vi "ImportedVideoConversion-CSV.vi"() -> ()   [LabVIEW 2019]
uses:
  RGB_To_Gray DLL Project/Project RGBToGray VI/RGBToGray.dll
  Gray_To_RGB DLL Project/Project Library For VI/Gray_to_RGB.dll
panel:
  out "Numeric":i32
  out "Frame Data":T1
  out "Elapsed time for Gray in sec":dbl
  out "RGB Frame":T2(plugin-control)
  out "Gray Frame":T2(plugin-control)
  in  "CSV File Path 2":path
  out "Elapsed time for RGB in sec":dbl
  out "Original Frame":T2(plugin-control)
  in  "Available Colormaps":T3
  in  "Stop":bool
  out "Progress Bar":i32(slide) max=677 scale=-1.0..677.0
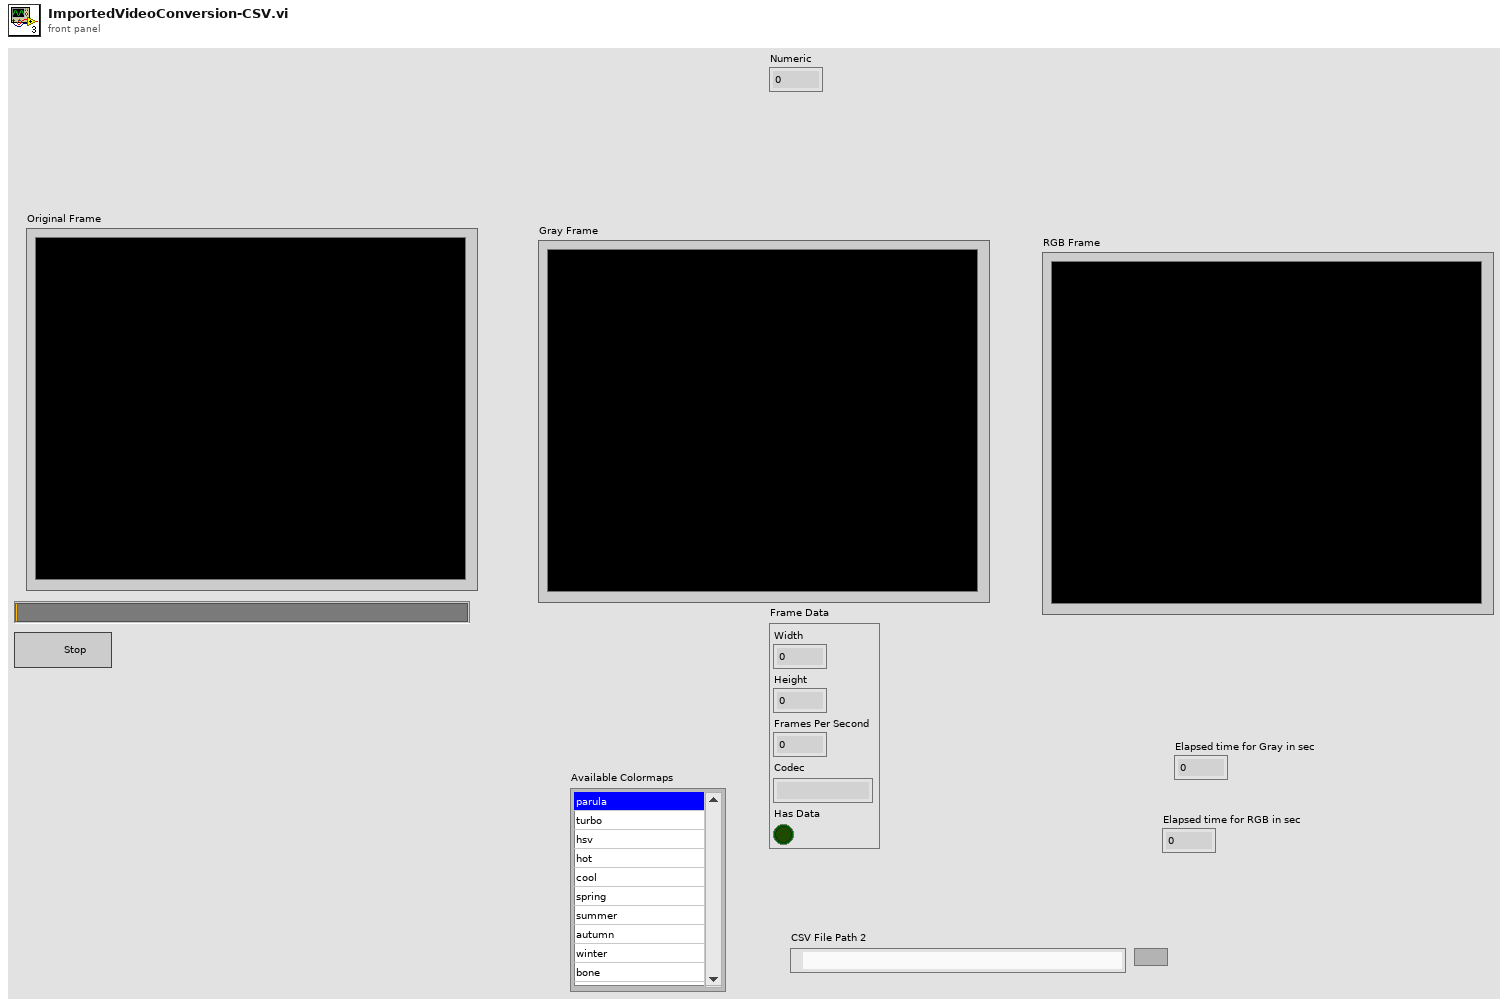
[diagram p1: front panel]
types:
  T1 = cluster{"Width":u32, "Height":u32, "Frames Per Second":u32, "Codec":string, "Has Data":bool}
  T2 = typedef "IMAQ Image.ctl" = refnum<image>
  T3 = typedef "Control 1.ctl" = i32
  T4 = typedef "Image Type" = u32
  T5 = typedef "IMAQ AVI2 Refnum.ctl" = refnum<k20>
  T6 = enum32{"Map Pixel Pointer", "Unmap Pixel Pointer", "Get Pixels Infos"}
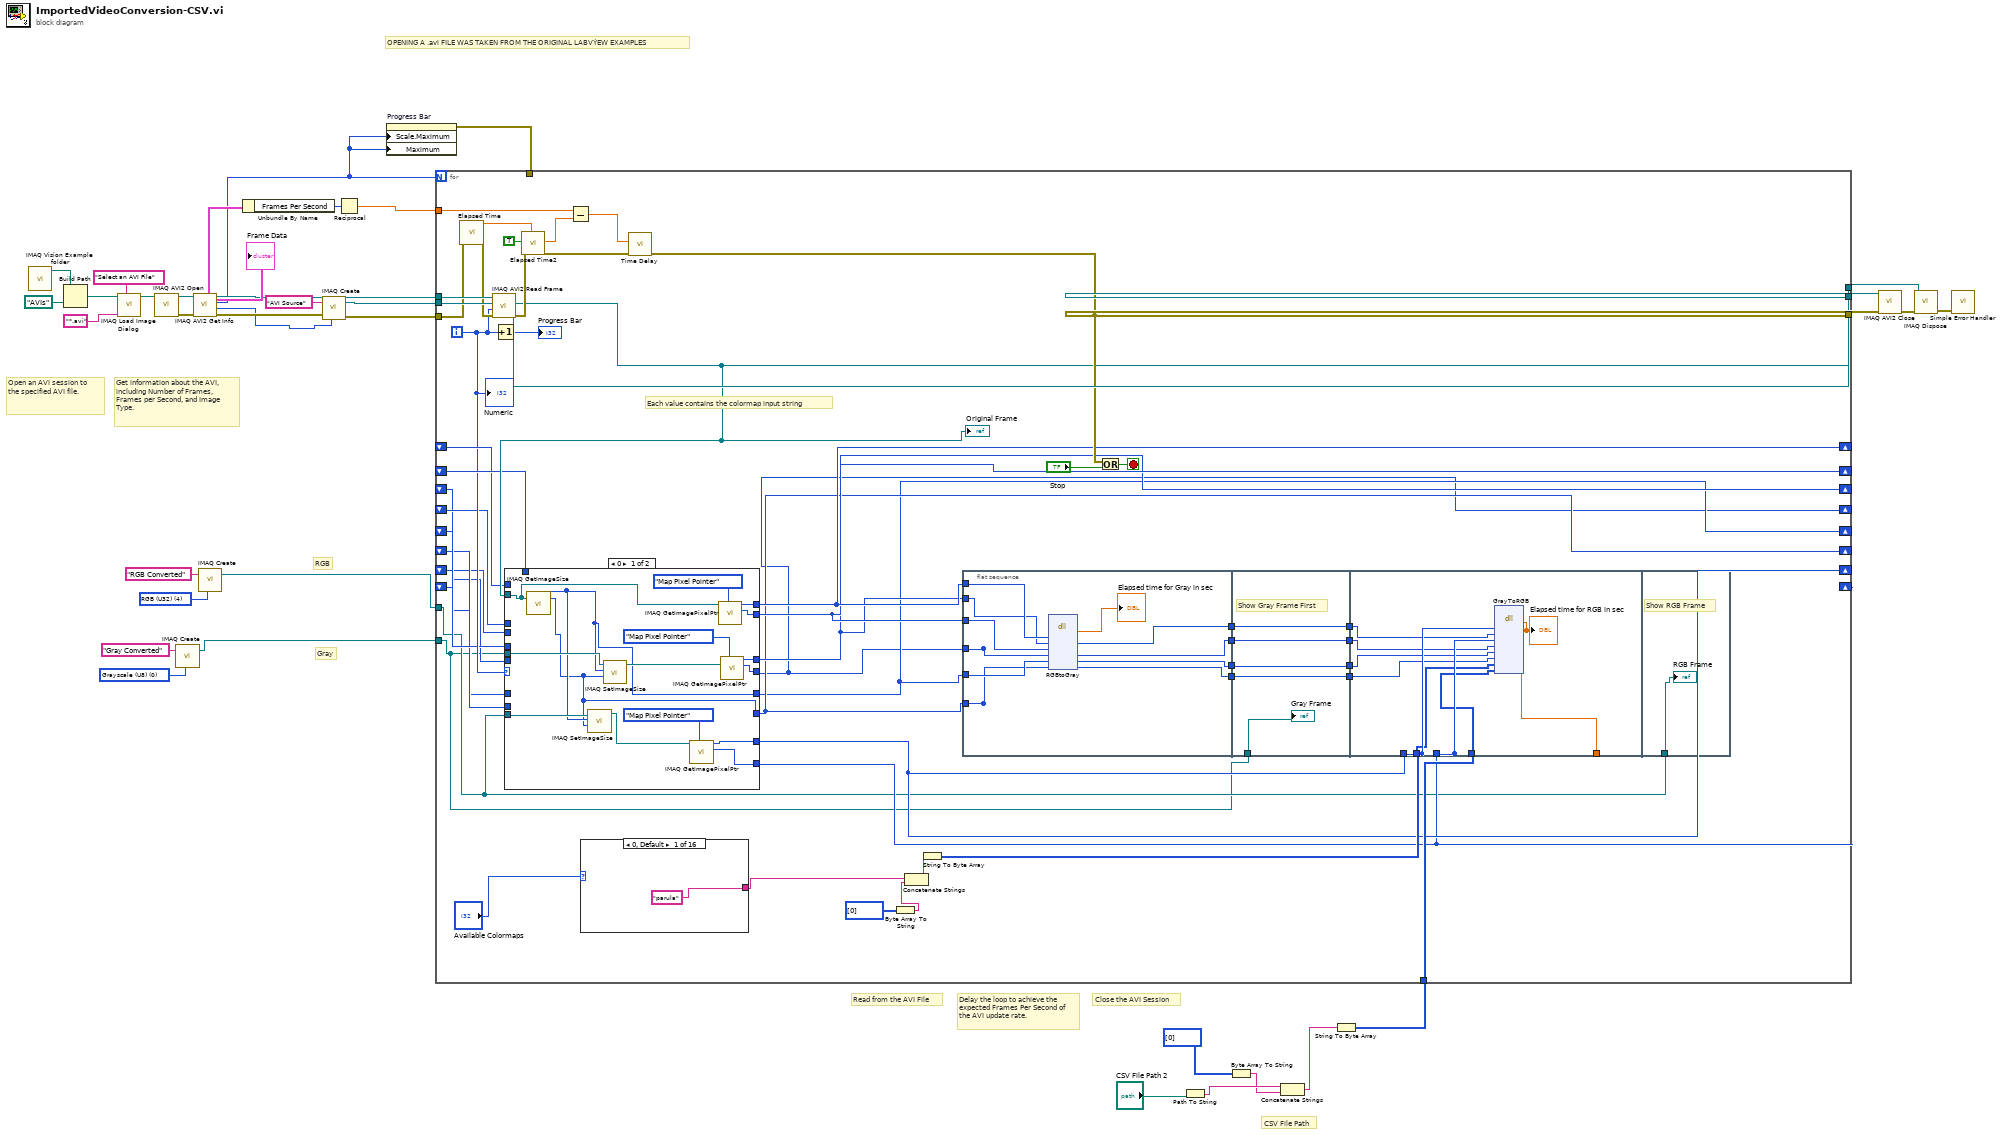
[diagram p0: block diagram]
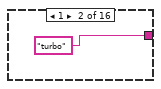
[diagram p3: hidden frame]
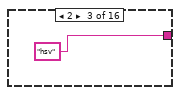
[diagram p4: hidden frame]
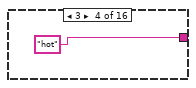
[diagram p5: hidden frame]
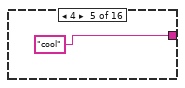
[diagram p6: hidden frame]
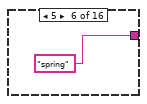
[diagram p7: hidden frame]
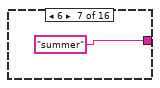
[diagram p8: hidden frame]
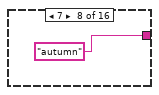
[diagram p9: hidden frame]
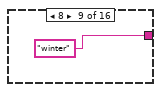
[diagram p10: hidden frame]
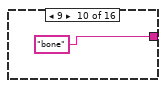
[diagram p11: hidden frame]
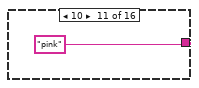
[diagram p12: hidden frame]
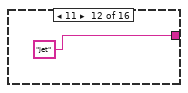
[diagram p13: hidden frame]
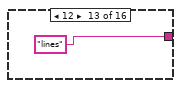
[diagram p14: hidden frame]
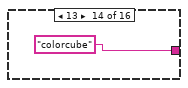
[diagram p15: hidden frame]
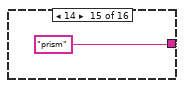
[diagram p16: hidden frame]
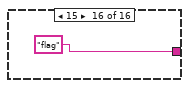
[diagram p17: hidden frame]
diagram:
  w8 = T4 0 items=["Grayscale (U8)", "Grayscale (I16)", "Grayscale (SGL)", "Complex (CSG)", "RGB (U32)", "HSL (U32)", "RGB (U64)", "Grayscale (U16)"] ("Image Type")
  w10 = T4 4 items=["Grayscale (U8)", "Grayscale (I16)", "Grayscale (SGL)", "Complex (CSG)", "RGB (U32)", "HSL (U32)", "RGB (U64)", "Grayscale (U16)"] ("Image Type")
  # "CSV File Path"
  # "Gray"
  # "RGB"
  # "OPENING A .avi FILE WAS TAKEN FROM THE ORIGINAL LABVÝEW EXAMPLES"
  # "Close the AVI Session"
  # "Read from the AVI File"
  # "Get information about the AVI, including Number of Frames, Frames per Second, and Image Type."
  # "Open an AVI session to the specified AVI file."
  # "Delay the loop to achieve the expected Frames Per Second of the AVI update rate."
  n1 = call "IMAQ Vision Example folder.vi"() -> ("Example Image Path"=w21:path)  [unwired: 11 in]
  n2 = Build Path(base path=w21, name or relative path=path "AVIs") -> (appended path=w18:path)
  n3 = call "IMAQ Load Image Dialog"("Prompt"="Select an AVI File" ("prompt"), "Pattern"="*.avi", "Start Path"=w18) -> ("Path"=w17:path)  [unwired: 6 in, 2 out]
  n4 = call "IMAQ AVI2 Open"("AVI File Path"=w17) -> ("error out"=w33:errorcluster, "AVI Refnum"=w32:T5)  [unwired: 2 in, 7 out]
  n5 = call "IMAQ Create"("Image Name"="Gray Converted", "Image Type"=w8) -> ("New Image"=w7:T2)  [unwired: 3 in, 1 out]
  n6 = call "IMAQ AVI2 Get Info"("error in (no error)"=w33, "AVI Refnum"=w32) -> ("error out"=w29:errorcluster, "Image Type"=w13:T4, "Number of Frames"=w15:u32, "AVI Refnum (duplicate)"=w26:T5, "Frame Data"=w34:T1)  [unwired: 5 out]
  "Frame Data" <- w34
  n7 = call "IMAQ Create"("Image Name"="RGB Converted", "Image Type"=w10) -> ("New Image"=w11:T2)  [unwired: 3 in, 1 out]
  n8 = Unbundle By Name(w34) -> ("Frames Per Second"=w23:u32)
  n9 = call "IMAQ Create"("Image Name"="AVI Source", "Image Type"=w13, "error in (no error)"=w29) -> ("New Image"=w27:T2, "error out"=w28:errorcluster)  [unwired: 1 in, 1 out]
  n10 = Reciprocal(x=w23) -> (1/x=w22:dbl)
  n11 = property on="Progress Bar" class="Slide (strict)"("Scale.Maximum"=w15, "Maximum"=w15) -> (error out=w14:errorcluster)  [unwired: 2 in, 1 out]
  n12 = Path To String(path="CSV File Path 2") -> (string=w4:string)
  n13 = Byte Array To String(unsigned byte array=u8[] [0]) -> (string=w3:string)
  n14 = Concatenate Strings(w4, w3) -> (w2:string)
  n15 = String To Byte Array(string=w2) -> (unsigned byte array=w1:u8[])
  n16 = for {
    N: w15 -> [_]
    tunnel: w27 -> [w86]
    tunnel: [w85] -> w30
    tunnel: [w75] -> w31
    tunnel: w28 -> [w84]
    tunnel: w26 -> [w87]
    tunnel: [w66] -> w24
    tunnel: w22 -> [w82]
    tunnel: w14 -> [_]
    tunnel: w11 -> [w40]
    tunnel: w7 -> [w39]
    shift-right: [w46] -> _
    shift-left: _ -> [w64]
    shift-right: [w45] -> _
    shift-left: _ -> [w65]
    shift-right: [w44] -> _
    shift-left: _ -> [w61]
    shift-right: [w41] -> _
    shift-left: _ -> [w62]
    shift-right: [w42] -> _
    shift-left: _ -> [w59]
    shift-right: [w43] -> _
    shift-left: _ -> [w60]
    shift-right: [w48] -> _
    shift-left: _ -> [w57]
    shift-right: [w47] -> _
    shift-left: _ -> [w58]
    tunnel: w1 -> [w50]
    i -> [w63]
    stop <- w73 stop-if-true
    # "Each value contains the colormap input string"
    n17 = call "Elapsed Time"("error in (no error)"=w84) -> ("Present (s)"=w80:dbl, "error out"=w83:errorcluster)  [unwired: 11 in, 6 out]
    n18 = call "IMAQ AVI2 Read Frame"("error in (no error)"=w83, "Frame Number"=w63, "Image"=w86, "AVI Refnum"=w87) -> ("error out"=w78:errorcluster, "Image Out"=w66:T2, "AVI Refnum (duplicate)"=w85:T5)  [unwired: 5 out]
    "Original Frame" <- w66
    n19 = Increment(x=w63) -> (x+1=→"Progress Bar":i32)
    n20 = case shown="0" w63 {
      tunnel: w66 -> [w118 _]
      tunnel: w39 -> [w124 _]
      tunnel: w40 -> [w123 _]
      tunnel: [w122 w131] -> w48
      tunnel: [w121 w130] -> w47
      tunnel: [w120 w135] -> w44
      tunnel: [w119 w134] -> w41
      tunnel: [w117 w133] -> w42
      tunnel: [w116 w132] -> w43
      tunnel: [w115 w137] -> w46
      tunnel: [w114 w136] -> w45
      tunnel: w64 -> [_ w137]
      tunnel: w65 -> [_ w136]
      tunnel: w61 -> [_ w135]
      tunnel: w62 -> [_ w134]
      tunnel: w59 -> [_ w133]
      tunnel: w60 -> [_ w132]
      tunnel: w57 -> [_ w131]
      tunnel: w58 -> [_ w130]
      frame 0 {
        n21 = call "IMAQ GetImageSize"("Image"=w118) -> ("Y Resolution"=w116:i32, "X Resolution"=w117:i32)  [unwired: 3 in, 1 out]
        n22 = call "IMAQ SetImageSize"("Y Resolution"=w116, "X Resolution"=w117, "Image"=w123) -> ("Image Out"=w127:T2)  [unwired: 2 in, 1 out]
        n23 = call "IMAQ SetImageSize"("Y Resolution"=w116, "X Resolution"=w117, "Image"=w124) -> ("Image Out"=w125:T2)  [unwired: 2 in, 1 out]
        n24 = call "IMAQ GetImagePixelPtr"("Function"=T6."Map Pixel Pointer", "Image"=w127) -> ("LineWidth(Pixels)"=w121:i32, "Pixel Pointer out"=w122:u64)  [unwired: 4 in, 4 out]
        n25 = call "IMAQ GetImagePixelPtr"("Function"=T6."Map Pixel Pointer", "Image"=w118) -> ("LineWidth(Pixels)"=w114:i32, "Pixel Pointer out"=w115:u64)  [unwired: 4 in, 4 out]
        n26 = call "IMAQ GetImagePixelPtr"("Function"=T6."Map Pixel Pointer", "Image"=w125) -> ("LineWidth(Pixels)"=w119:i32, "Pixel Pointer out"=w120:u64)  [unwired: 4 in, 4 out]
      }
      frame 1, Default {
      }
    }
    n27 = call "Elapsed Time2"("Reset"=TRUE, "error in (no error)"=w78, "Set Start Time (s)"=w80) -> ("Elapsed Time (s)"=w77:dbl, "error out"=w76:errorcluster)  [unwired: 9 in, 6 out]
    n28 = Subtract(x=w82, y=w77) -> (x-y=w81:dbl)
    n29 = case shown="0, Default" "Available Colormaps" {
      tunnel: ["parula" "turbo" "hsv" "hot" "cool" "spring" "summer" "autumn" "winter" "bone" "pink" "jet" "lines" "colorcube" "prism" "flag"] -> w67
      frame 0, Default {
      }
      frame 1 {
      }
      frame 2 {
      }
      frame 3 {
      }
      frame 4 {
      }
      frame 5 {
      }
      frame 6 {
      }
      frame 7 {
      }
      frame 8 {
      }
      frame 9 {
      }
      frame 10 {
      }
      frame 11 {
      }
      frame 12 {
      }
      frame 13 {
      }
      frame 14 {
      }
      frame 15 {
      }
    }
    n30 = call "Time Delay"("error in (no error)"=w76, "Delay Time (s)"=w81) -> ("error out"=w75:errorcluster)  [unwired: 9 in]
    n31 = Byte Array To String(unsigned byte array=u8[] [0]) -> (string=w69:string)
    n32 = Concatenate Strings(w67, w69) -> (w68:string)
    n33 = String To Byte Array(string=w68) -> (unsigned byte array=w49:u8[])
    n34 = flat-sequence {
      tunnel: [w91] -> w56
      tunnel: [w90] -> w55
      tunnel: w46 -> [w98]
      tunnel: w44 -> [w97]
      tunnel: w45 -> [w96]
      tunnel: w41 -> [w95]
      tunnel: w42 -> [w94]
      tunnel: [w93] -> _
      tunnel: [w95] -> _
      tunnel: w43 -> [w93]
      tunnel: [w89] -> w38
      tunnel: [w88] -> w37
      tunnel: w56 -> [w103]
      tunnel: [w103] -> w54
      tunnel: w55 -> [w102]
      tunnel: [w102] -> w53
      tunnel: [w101] -> w52
      tunnel: [w100] -> w51
      tunnel: w39 -> [w99]
      tunnel: w38 -> [w101]
      tunnel: w37 -> [w100]
      tunnel: w49 -> [w106]
      tunnel: w50 -> [w105]
      tunnel: w54 -> [w111]
      tunnel: w53 -> [w109]
      tunnel: w52 -> [w108]
      tunnel: w51 -> [w107]
      tunnel: [w112] -> _
      tunnel: [w110] -> _
      tunnel: [w104] -> _
      tunnel: w48 -> [w112]
      tunnel: w47 -> [w110]
      tunnel: w40 -> [w113]
      frame #0 {
        n35 = dll-call lib="C:/Users/byald/Desktop/EE-433 Project Group1/RGB_To_Gray DLL Project/Project RGBToGray VI/RGBToGray.dll" fn="RGBtoGray"("RGBImage"=w98, "GrayImage"=w97, "LVLineWidthRGB"=w96, "LVLineWidthGray"=w95, "LVWidth"=w94, "LVHeight"=w93) -> ("return type"=→"Elapsed time for Gray in sec":dbl, "GrayImage"=w91:u64, "LVLineWidthGray"=w90:i32, "LVWidth"=w89:i32, "LVHeight"=w88:i32)  [unwired: 5 in, 2 out]
      }
      frame #1 {
        # "Show Gray Frame First"
        "Gray Frame" <- w99
      }
      frame #2 {
        n36 = dll-call lib="C:/Users/byald/Desktop/EE-433 Project Group1/Gray_To_RGB DLL Project/Project Library For VI/Gray_to_RGB.dll" fn="GrayToRGB"("RGBImage"=w112, "GrayImage"=w111, "LVLineWidthRGB"=w110, "LVLineWidthGray"=w109, "LVWidth"=w108, "LVHeight"=w107, "ColorMap"=w106, "CsvPath"=w105) -> ("return type"=w104:dbl)  [unwired: 11 in, 2 out]
        "Elapsed time for RGB in sec" <- w104
      }
      frame #3 {
        # "Show RGB Frame"
        "RGB Frame" <- w113
      }
    }
    n37 = Or(x=w75, y="Stop") -> (x .or. y?=w73:bool)
    "Numeric" <- w63
  }
  n38 = call "IMAQ AVI2 Close"("error in (no error)"=w31, "AVI Refnum"=w30) -> ("error out"=w25:errorcluster)  [unwired: 9 out]
  n39 = call "IMAQ Dispose"("Image"=w24, "error in (no error)"=w25) -> ("error out"=w35:errorcluster)  [unwired: 1 in, 3 out]
  n40 = call <vilib>:"Simple Error Handler.vi"("error in (no error)"=w35) -> ()  [unwired: 1 in, 8 out]
